vi "Process.vi"(8 "error in":errorcluster, 11 "EmbeddedSMO":refnum<class "SMO.UI.Embedded.lvclass">) -> (0 "error out":errorcluster, 3 "EmbeddedSMO out":refnum<class "SMO.UI.Embedded.lvclass">)   [LabVIEW 2019, in "SMO.UI.Embedded.lvclass"]
doc: "---------------------------------------------------------------\nJKI State Machine Objects™\nhttp://jki.net/state-machine-objects/\nCopyright (C) 2005-2015, JKI <info@jki.net>\nALL RIGHTS RESERVEDJKI State Machine Objects (SMO) 1.0.0.5\nJKI - JKI\nCopyright (c) 2016, JKI"
uses:
  SMO.UI.Embedded.lvclass
  C:/Program Files (x86)/National Instruments/LabVIEW 2019/vi.lib/JKI/JKI SMO/SMO/SMO.lvclass
  C:/Program Files (x86)/National Instruments/LabVIEW 2019/vi.lib/JKI/JKI SMO/SMO.UI/SMO.UI.lvclass
  <vilib>/JKI/JKI SMO/SMO/Typedefs/Parent Call--Enum.ctl
  SMO.UI.Embedded.lvclass/SMO.UI.Embedded.ctl
  <vilib>/JKI/JKI SMO/SMO/SMO.lvclass/SMO.ctl
  <vilib>/JKI/JKI SMO/SMO/Private/ReftoDVR--SMO.vi
  <vilib>/JKI/JKI SMO/SMO.UI/SMO.UI.lvclass
  <vilib>/JKI/JKI SMO/SMO/SMO.lvclass
panel:
  # "For instructions on how to use the JKI State Machine Objects, examples and video tutorials, visit:\nhttp://jki.net/state-machine-objects/\n\nJKI State Machine Objects™\nhttp://jki.net/state-machine-objects/\nCopyright (C) 2005-2015, JKI <info@jki.net>\nALL RIGHTS RESERVED"
  # "SMO UI Template"
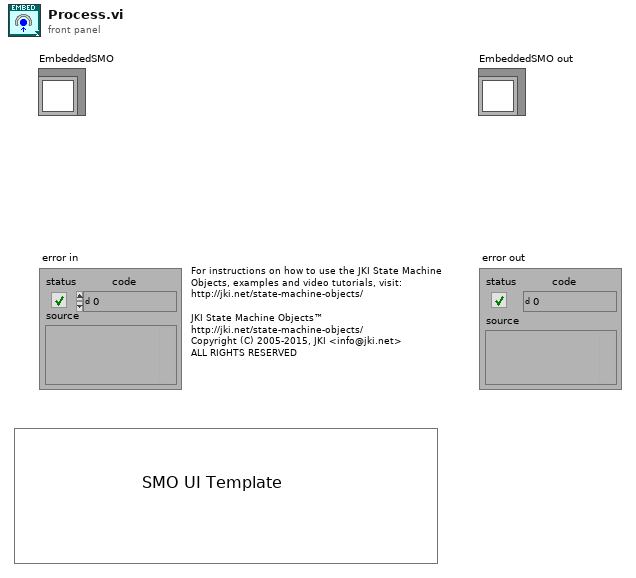
[diagram p1: front panel]
types:
  T1 = typedef "SMO.lvclass/Parent Call--Enum.ctl" = enum16{"Allows parent to run", "Does not request parent to run"}
  T2 = enum32{"invalid app kind", "Development System", "Run Time System", "Student Edition", "Embedded LabVIEW", "Evaluation", "Custom"}
  T3 = enum32{"Invalid", "Standard", "Closed", "Hidden", "Minimized", "Maximized"}
  T4 = typedef "SMO.UI.Embedded.lvclass/PrivateEvents--EmbeddedSMO.WriteName.ctl" = string
  T5 = cluster{"Core":cluster{"Current VI Reference":refnum<vi>, "Close Panel on Exit?":bool, "error":errorcluster}, "Self":refnum<class "SMO.UI.Embedded.lvclass">, "Your string data":string}
  T6 = typedef "SMO.UI.Embedded.lvclass/PrivateEvents--EmbeddedSMO.GetName.ctl" = refnum<notifier>
  T7 = typedef "SMO.UI.Embedded.lvclass/GetUIStateNotifier.ctl" = refnum<notifier>
  T8 = typedef "SMO.UI.Embedded.lvclass/UI State.ctl" = enum16{"unknown", "Opened", "Embedded", "Closed"}
  T9 = typedef "SMO.UI.Embedded.lvclass/PrivateEvents--EmbeddedSMO.GetSubPanelReference.ctl" = refnum<notifier>
  T10 = typedef "SMO.UI.Embedded.lvclass/PrivateEvents--EmbeddedSMO.SetSubpanelReference.ctl" = refnum<vi>
  T11 = cluster{"Current VI Reference":refnum<vi>, "Close Panel on Exit?":bool, "error":errorcluster}
  T12 = typedef "SMO.UI.Embedded.lvclass/PrivateEvents--Cluster.ctl" = cluster{"Get UI State":refnum<user-event>, "SetUIState":refnum<user-event>, "GetSubPanelReference":refnum<user-event>, "SetSubpanelReference":refnum<user-event>, "WriteName":refnum<user-event>, "GetName":refnum<user-event>}
  T13 = typedef "SMO.lvclass/Protected Events.ctl" = cluster{"StopProcesses":refnum<user-event>, "AbortProcesses":refnum<user-event>, "Config Changed":refnum<user-event>, "Dependency":refnum<user-event>}
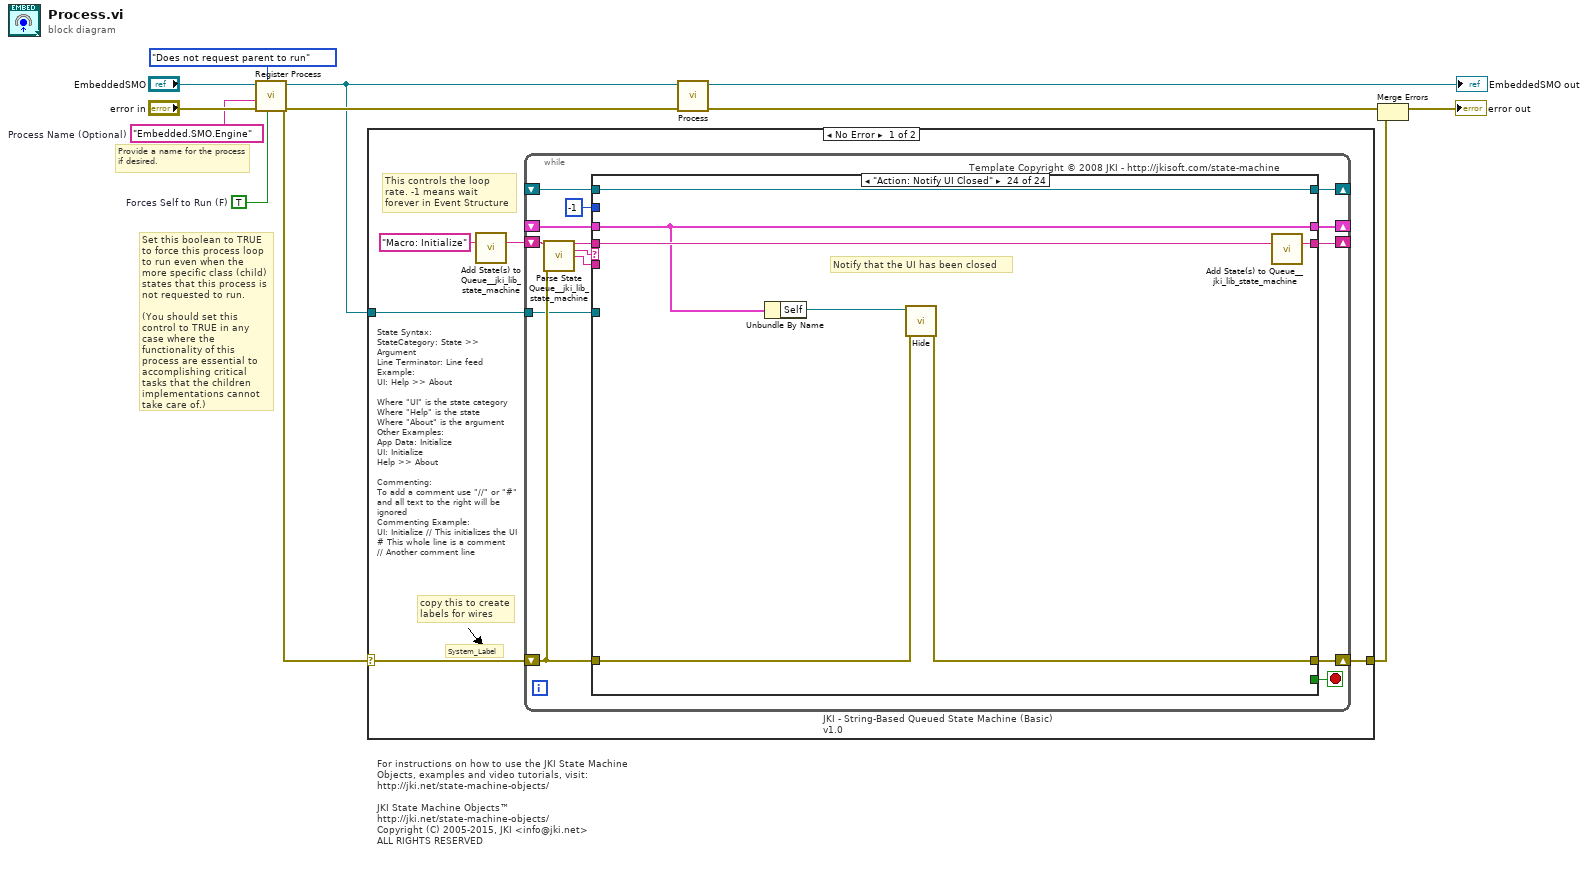
[diagram p0: block diagram]
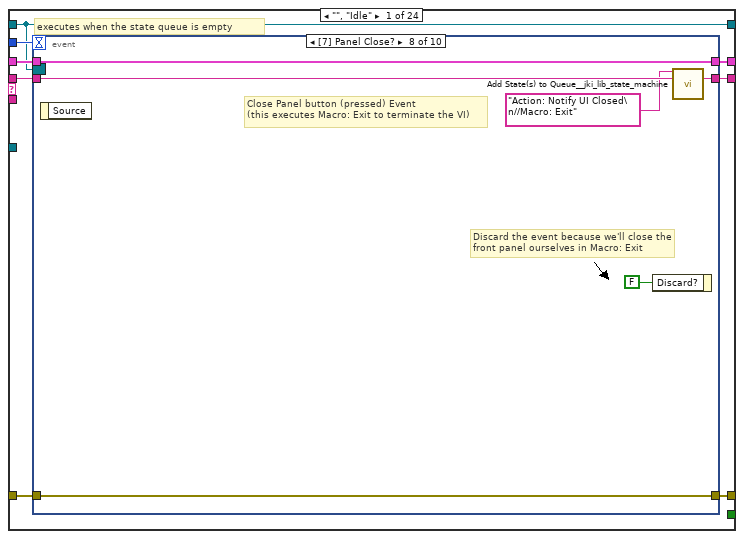
[diagram p2: hidden frame]
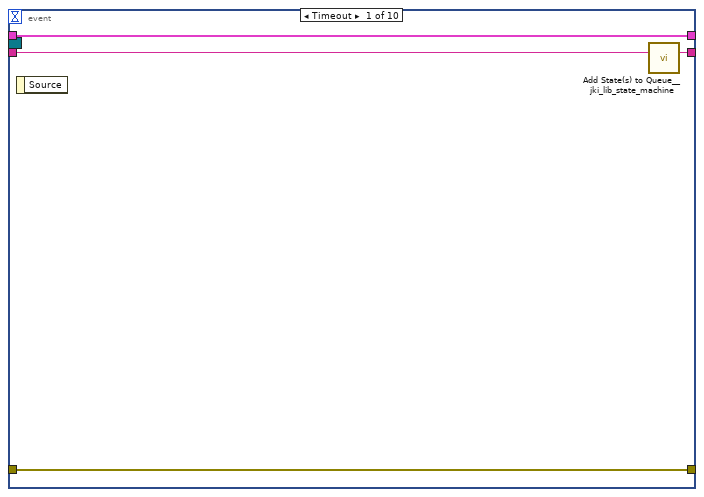
[diagram p3: hidden frame]
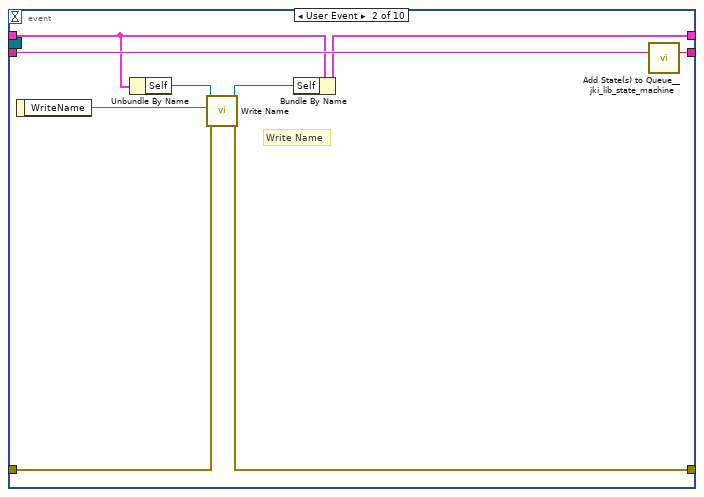
[diagram p4: hidden frame]
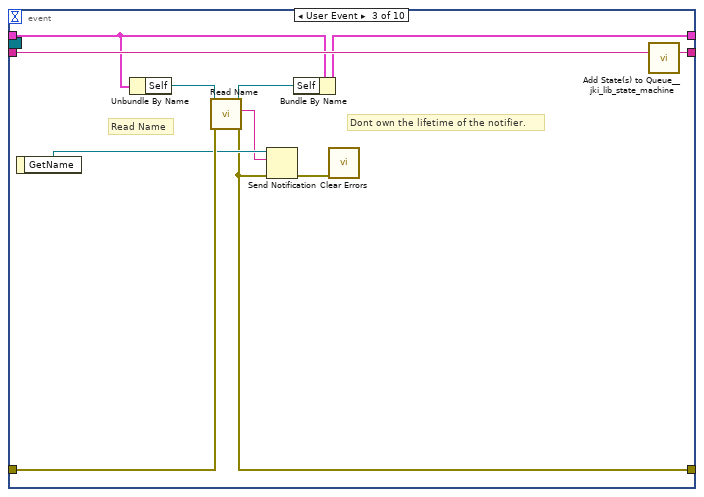
[diagram p5: hidden frame]
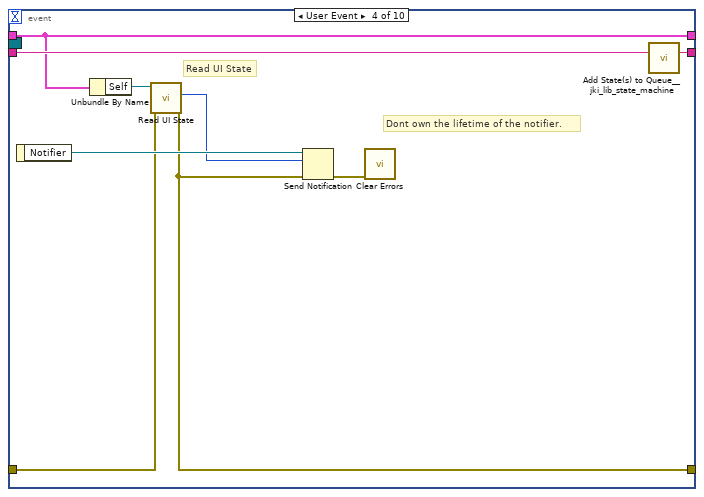
[diagram p6: hidden frame]
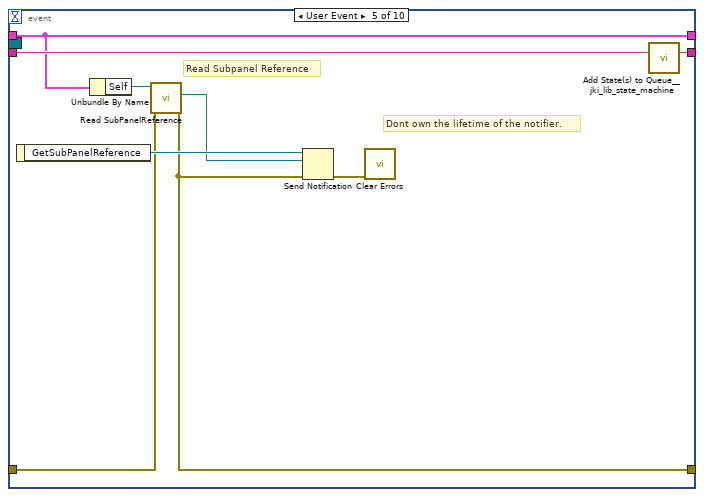
[diagram p7: hidden frame]
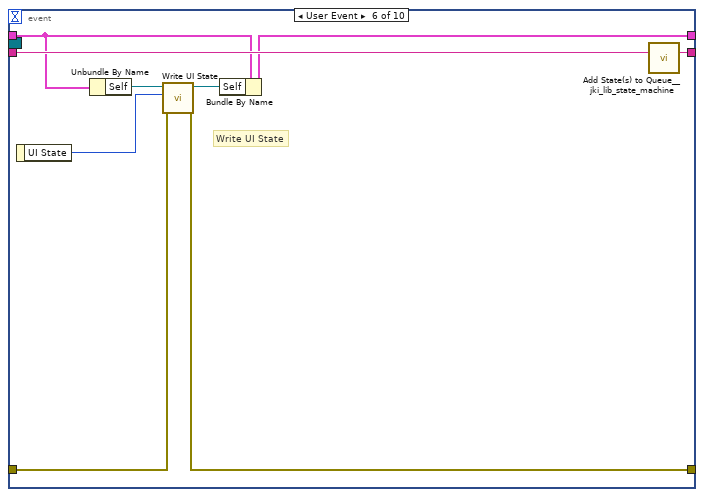
[diagram p8: hidden frame]
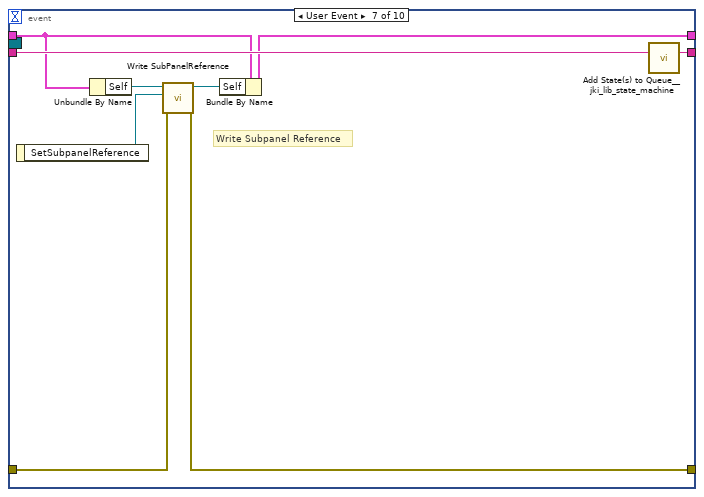
[diagram p9: hidden frame]
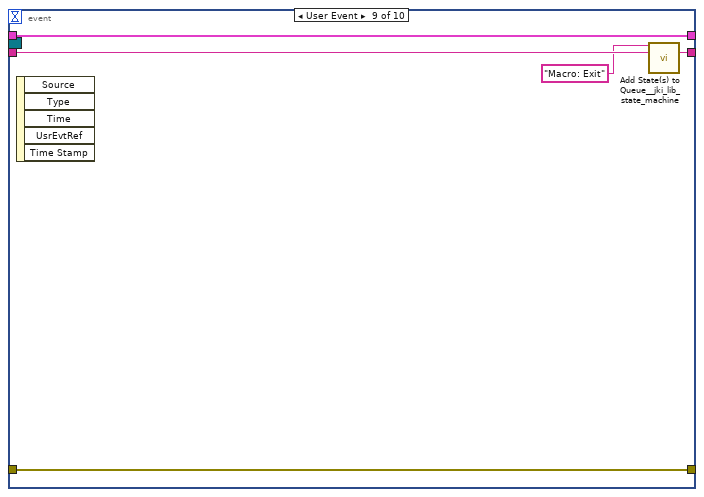
[diagram p10: hidden frame]
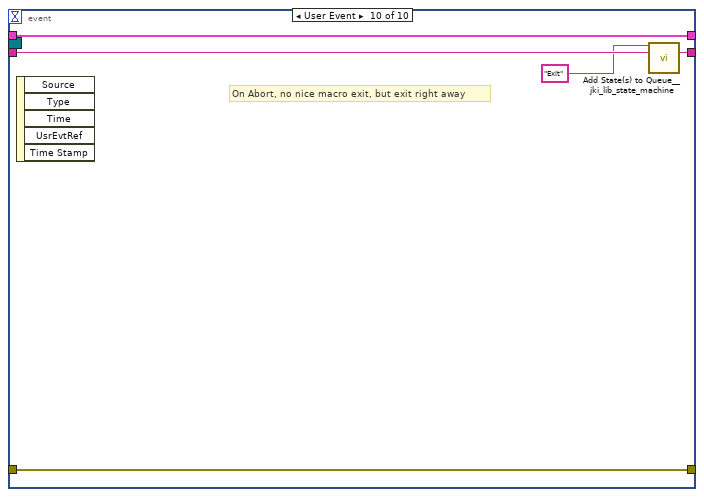
[diagram p11: hidden frame]
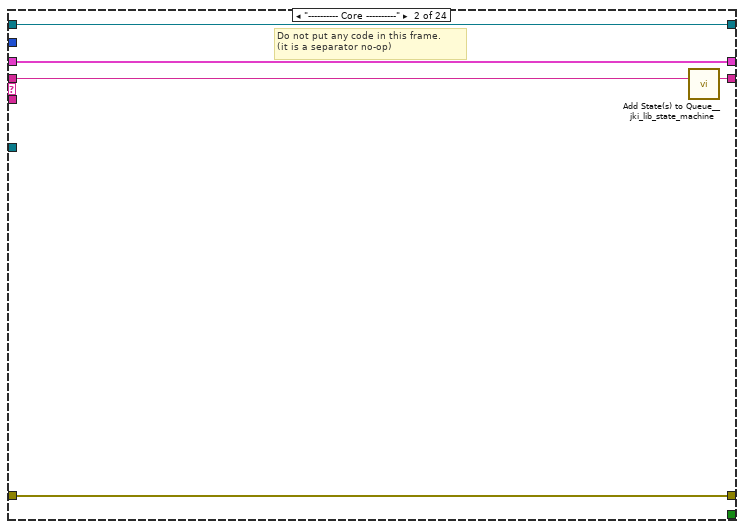
[diagram p12: hidden frame]
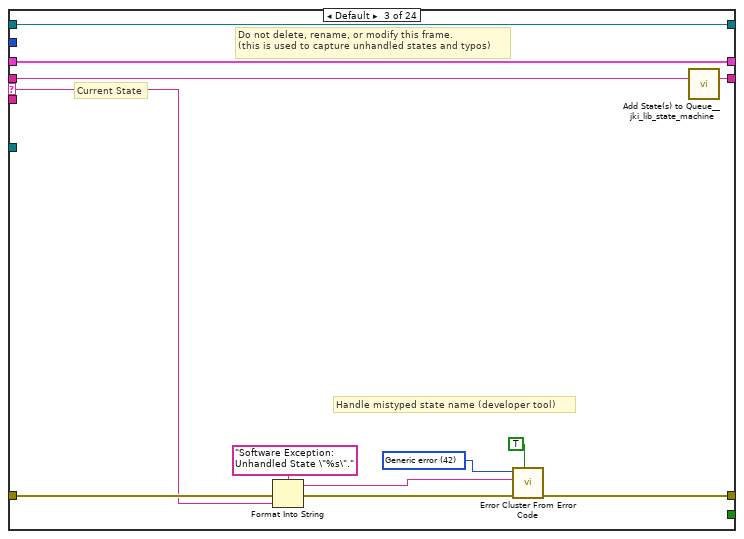
[diagram p13: hidden frame]
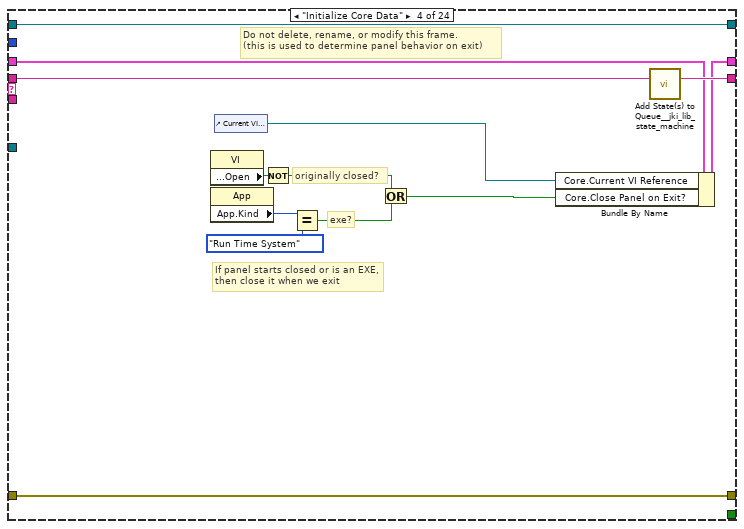
[diagram p14: hidden frame]
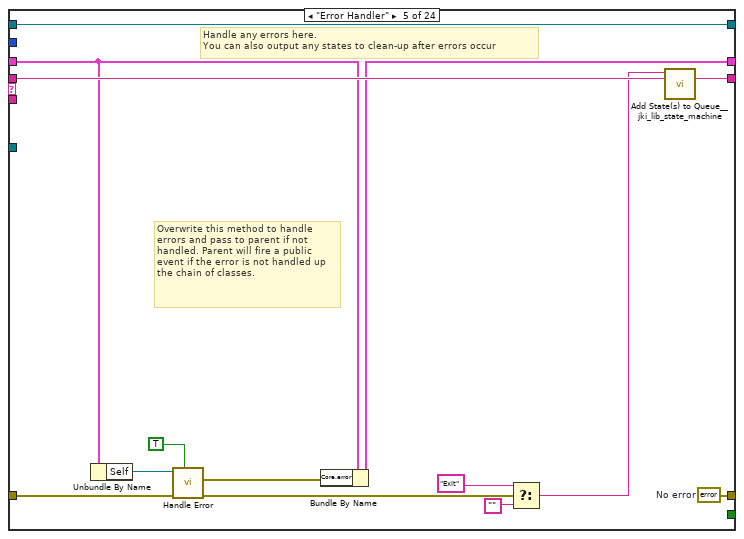
[diagram p15: hidden frame]
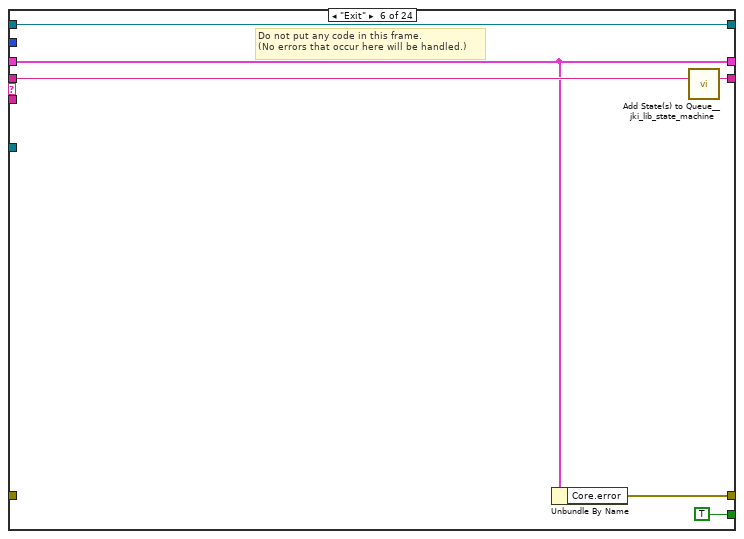
[diagram p16: hidden frame]
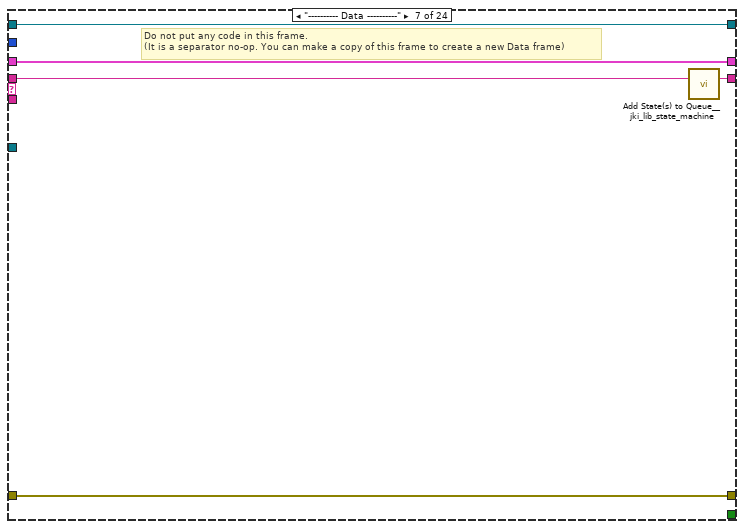
[diagram p17: hidden frame]
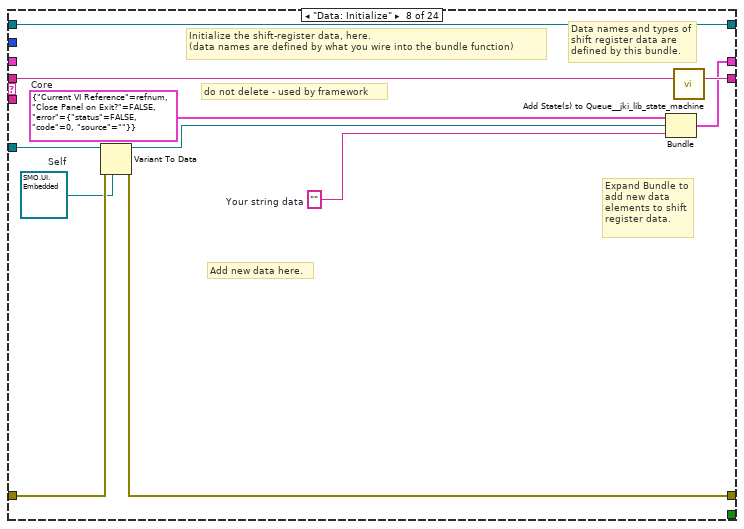
[diagram p18: hidden frame]
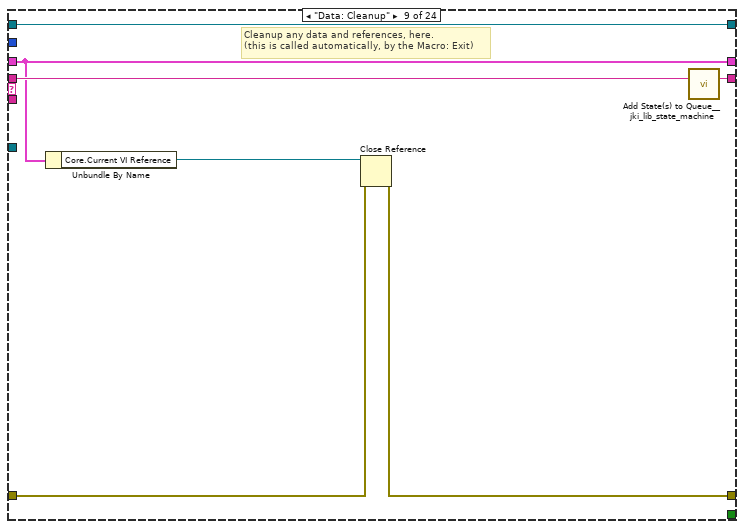
[diagram p19: hidden frame]
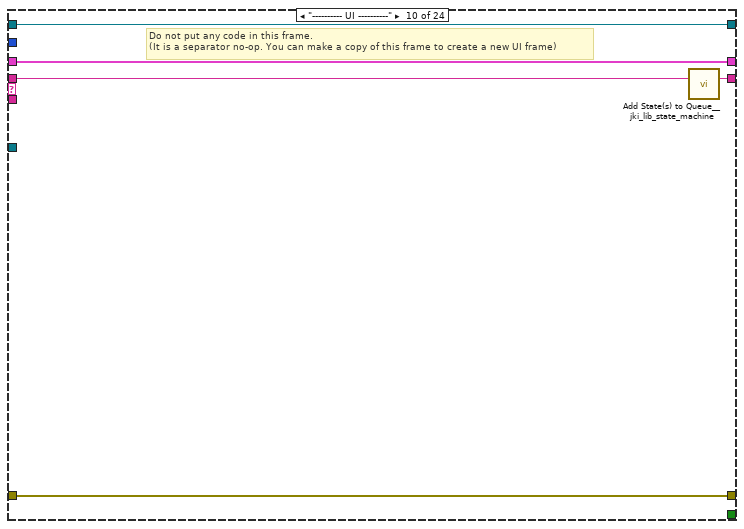
[diagram p20: hidden frame]
diagram:
  w2 = TRUE  # Forces Self to Run (F)
  w1 = "Embedded.SMO.Engine"  # Process Name (Optional)
  # "Provide a name for the process\nif desired."
  # "Set this boolean to TRUE to force this process loop to run even when the more specific class (child) states that this process is not requested to run.\n\n(You should set this control to TRUE in any case where the functionality of this process are essential to accomplishing critical tasks that the children implementations cannot take care of.)"
  # "For instructions on how to use the JKI State Machine Objects, examples and video tutorials, visit:\nhttp://jki.net/state-machine-objects/\n\nJKI State Machine Objects™\nhttp://jki.net/state-machine-objects/\nCopyright (C) 2005-2015, JKI <info@jki.net>\nALL RIGHTS RESERVED"
  n1 = call <vilib>:"Register Process.vi"("Forces Self to Run (F)"=w2, "Parent Call"=Parent_Call--Enum."Does not request parent to run", "error in (no error)"="error in", "Process Name (optional)"=w1, "SMO"="EmbeddedSMO") -> ("error out"=w8:errorcluster, "SMO out"=w7:refnum<class "SMO.UI.Embedded.lvclass">)  [unwired: 5 in]
  n2 = case shown="No Error" w8 {
    selector: w8 -> [w13 w342]
    tunnel: w7 -> [w14 _]
    tunnel: [w12 w342] -> w4
    frame No Error {
      # "State Syntax:\nStateCategory: State >> Argument\nLine Terminator: Line feed\nExample:\nUI: Help >> About\n\nWhere \"UI\" is the state category\nWhere \"Help\" is the state\nWhere \"About\" is the argument\nOther Examples:\nApp Data: Initialize\nUI: Initialize\nHelp >> About\n\nCommenting:\nTo add a comment use \"//\" or \"#\" and all text to the right will be ignored\nCommenting Example:\nUI: Initialize // This initializes the UI\n# This whole line is a comment\n// Another comment line"
      # "copy this to create labels for wires"
      # "This controls the loop rate. -1 means wait forever in Event Structure"
      # "System_Label"
      n3 = call <vilib>:"Add State(s) to Queue__jki_lib_state_machine.vi"("State(s) in (\"\")"="Macro: Initialize") -> ("States Out"=w16:string)  [unwired: 14 in]
      n4 = while "JKI - String-Based Queued State Machine (Basic) v1.0" {
        shift-right: [w23] -> _
        shift-left: _ -> [w22]
        shift-right: [w26] -> w12
        shift-left: w13 -> [w20]
        shift-right: [w25] -> _
        shift-left: w16 -> [w27]
        tunnel: w14 -> [w19]
        shift-right: [w18] -> _
        shift-left: _ -> [w17]
        stop <- w24 stop-if-true
        # "Template Copyright © 2008 JKI - http://jkisoft.com/state-machine"
        n5 = call <vilib>:"Parse State Queue__jki_lib_state_machine.vi"("State Queue"=w27, "Error In (no error)"=w20) -> ("Remaining States"=w29:string, "Current State"=w30:string, "Arguments"=w28:string)  [unwired: 11 in]
        n6 = case shown="\"Action: Notify UI Closed\"" w30 {
          selector: w30 -> [_ _ w121 _ _ _ _ _ _ _ _ _ _ _ _ _ _ _ _ _ _ _ _ _]
          tunnel: w29 -> [w38 w119 w125 w144 w158 w164 w169 w180 w187 w192 w200 w207 w223 w255 w264 w278 w283 w294 w299 w311 w317 w324 w334 w341]
          tunnel: w28 -> [_ _ _ _ _ _ _ _ _ _ _ w201 w217 _ _ _ _ _ _ _ _ _ _ _]
          tunnel: w22 -> [w36 w116 w123 w135 w147 w160 w166 _ w182 w189 w196 w205 w219 w252 w260 w269 w280 w291 w296 w309 w315 w320 w331 w337]
          tunnel: [w35 w117 w127 w141 w149 w159 w167 w175 w183 w190 w198 w202 w220 w253 w262 w276 w281 w285 w297 w304 w312 w321 w325 w335] -> w26
          tunnel: w20 -> [w34 w117 w126 w141 w154 _ w167 w176 w184 w190 w198 w203 w221 w253 w262 w276 w281 w286 w297 w306 w313 w321 w326 w336]
          tunnel: [w37 w118 w124 w143 w157 w163 w168 w179 w186 w191 w199 w206 w222 w254 w263 w277 w282 w293 w298 w310 w316 w323 w333 w340] -> w25
          tunnel: [_ _ _ _ _ TRUE _ _ _ _ _ _ _ _ _ _ _ _ _ _ _ _ _ _] -> w24
          tunnel: [w33 w116 w123 w142 w146 w160 w166 w178 w182 w189 w196 w205 w219 w252 w260 w269 w280 w291 w296 w309 w315 w319 w330 w337] -> w23
          tunnel: -1 ("Timeout") -> [w32 _ _ _ _ _ _ _ _ _ _ _ _ _ _ _ _ _ _ _ _ _ _ _]
          tunnel: w19 -> [_ _ _ _ _ _ _ w173 _ _ _ _ _ _ _ _ _ _ _ _ _ _ _ _]
          tunnel: [w31 w115 w120 w132 w156 w161 w165 w171 w181 w188 w197 w204 w216 w251 w261 w270 w279 w292 w295 w308 w314 w322 w332 w339] -> w18
          tunnel: w17 -> [w31 w115 w120 w132 w156 w161 w165 w171 w181 w188 w197 w204 w216 w251 w261 w270 w279 w292 w295 _ w314 w322 w332 w339]
          frame "", "Idle" {
            # "executes when the state queue is empty"
            n7 = event shown="[7] Panel Close?" {
              selector: w31 -> [_ _ _ _ _ _ _ _ _ _]
              dyn-events: _ -> [_ _ _ _ _ _ _ _ _ _]
              timeout: w32 -> [_ _ _ _ _ _ _ _ _ _]
              tunnel: w38 -> [w42 w51 w62 w71 w80 w89 w98 w104 w109 w114]
              tunnel: [w41 w50 w61 w70 w79 w88 w97 w103 w108 w113] -> w37
              tunnel: w36 -> [w39 w48 w60 w69 w78 w83 w93 w100 w106 w111]
              tunnel: [w40 w45 w52 w63 w72 w84 w94 w99 w107 w112] -> w35
              tunnel: w34 -> [w40 w46 w56 w66 w73 w85 w95 w99 w107 w112]
              tunnel: [w39 w47 w59 w69 w78 w82 w92 w100 w106 w111] -> w33
              event Timeout {
                n8 = event-data() -> ()  [unwired: 1 in, 1 out]
                n9 = call <vilib>:"Add State(s) to Queue__jki_lib_state_machine.vi"("State(s) in (\"\")"=w42) -> ("States Out"=w41:string)  [unwired: 14 in]
              }
              event User Event {
                # "Write Name"
                n10 = event-data() -> ("WriteName"=w49:T4)  [unwired: 1 in]
                n11 = Unbundle By Name(w48) -> ("Self"=w44:refnum<class "SMO.UI.Embedded.lvclass">)
                n12 = call "Write Name.vi"("error in (no error)"=w46, "Name"=w49, "EmbeddedSMO in"=w44) -> ("error out"=w45:errorcluster, "EmbeddedSMO out"=w43:refnum<class "SMO.UI.Embedded.lvclass">)  [unwired: 7 in]
                n13 = Bundle By Name(cluster=w48, "Self"=w43) -> (w47:T5)
                n14 = call <vilib>:"Add State(s) to Queue__jki_lib_state_machine.vi"("State(s) in (\"\")"=w51) -> ("States Out"=w50:string)  [unwired: 14 in]
              }
              event User Event {
                # "Dont own the lifetime of the notifier."
                # "Read Name"
                n15 = event-data() -> ("GetName"=w54:T6)  [unwired: 1 in]
                n16 = Unbundle By Name(w60) -> ("Self"=w58:refnum<class "SMO.UI.Embedded.lvclass">)
                n17 = call "Read Name.vi"("error in (no error)"=w56, "EmbeddedSMO in"=w58) -> ("error out"=w52:errorcluster, "Name"=w53:string, "EmbeddedSMO out"=w57:refnum<class "SMO.UI.Embedded.lvclass">)  [unwired: 7 in]
                n18 = Send Notification(notification=w53, notifier=w54, error in (no error)=w52) -> (error out=w55:errorcluster)  [unwired: 1 out]
                n19 = Bundle By Name(cluster=w60, "Self"=w57) -> (w59:T5)
                n20 = call <vilib>:"Clear Errors.vi"("error in (no error)"=w55) -> ()  [unwired: 5 in, 2 out]
                n21 = call <vilib>:"Add State(s) to Queue__jki_lib_state_machine.vi"("State(s) in (\"\")"=w62) -> ("States Out"=w61:string)  [unwired: 14 in]
              }
              event User Event {
                # "Dont own the lifetime of the notifier."
                # "Read UI State"
                n22 = event-data() -> ("Notifier"=w68:T7)  [unwired: 1 in]
                n23 = Unbundle By Name(w69) -> ("Self"=w67:refnum<class "SMO.UI.Embedded.lvclass">)
                n24 = call "Read UI State.vi"("error in (no error)"=w66, "EmbeddedSMO in"=w67) -> ("error out"=w63:errorcluster, "UI State"=w65:T8)  [unwired: 7 in, 1 out]
                n25 = Send Notification(notification=w65, notifier=w68, error in (no error)=w63) -> (error out=w64:errorcluster)  [unwired: 1 out]
                n26 = call <vilib>:"Clear Errors.vi"("error in (no error)"=w64) -> ()  [unwired: 5 in, 2 out]
                n27 = call <vilib>:"Add State(s) to Queue__jki_lib_state_machine.vi"("State(s) in (\"\")"=w71) -> ("States Out"=w70:string)  [unwired: 14 in]
              }
              event User Event {
                # "Dont own the lifetime of the notifier."
                # "Read Subpanel Reference"
                n28 = event-data() -> ("GetSubPanelReference"=w77:T9)  [unwired: 1 in]
                n29 = Unbundle By Name(w78) -> ("Self"=w75:refnum<class "SMO.UI.Embedded.lvclass">)
                n30 = call "Read SubPanelReference.vi"("error in (no error)"=w73, "EmbeddedSMO in"=w75) -> ("error out"=w72:errorcluster, "SubPanelReference"=w74:refnum<vi>)  [unwired: 7 in, 1 out]
                n31 = Send Notification(notification=w74, notifier=w77, error in (no error)=w72) -> (error out=w76:errorcluster)  [unwired: 1 out]
                n32 = call <vilib>:"Clear Errors.vi"("error in (no error)"=w76) -> ()  [unwired: 5 in, 2 out]
                n33 = call <vilib>:"Add State(s) to Queue__jki_lib_state_machine.vi"("State(s) in (\"\")"=w80) -> ("States Out"=w79:string)  [unwired: 14 in]
              }
              event User Event {
                # "Write UI State"
                n34 = event-data() -> ("UI State"=w86:T8)  [unwired: 1 in]
                n35 = Unbundle By Name(w83) -> ("Self"=w87:refnum<class "SMO.UI.Embedded.lvclass">)
                n36 = call "Write UI State.vi"("error in (no error)"=w85, "UI State"=w86, "EmbeddedSMO in"=w87) -> ("error out"=w84:errorcluster, "EmbeddedSMO out"=w81:refnum<class "SMO.UI.Embedded.lvclass">)  [unwired: 7 in]
                n37 = Bundle By Name(cluster=w83, "Self"=w81) -> (w82:T5)
                n38 = call <vilib>:"Add State(s) to Queue__jki_lib_state_machine.vi"("State(s) in (\"\")"=w89) -> ("States Out"=w88:string)  [unwired: 14 in]
              }
              event User Event {
                # "Write Subpanel Reference"
                n39 = event-data() -> ("SetSubpanelReference"=w90:T10)  [unwired: 1 in]
                n40 = Unbundle By Name(w93) -> ("Self"=w96:refnum<class "SMO.UI.Embedded.lvclass">)
                n41 = call "Write SubPanelReference.vi"("error in (no error)"=w95, "SubPanelReference"=w90, "EmbeddedSMO in"=w96) -> ("error out"=w94:errorcluster, "EmbeddedSMO out"=w91:refnum<class "SMO.UI.Embedded.lvclass">)  [unwired: 7 in]
                n42 = Bundle By Name(cluster=w93, "Self"=w91) -> (w92:T5)
                n43 = call <vilib>:"Add State(s) to Queue__jki_lib_state_machine.vi"("State(s) in (\"\")"=w98) -> ("States Out"=w97:string)  [unwired: 14 in]
              }
              event Panel Close? {
                # "Discard the event because we'll close the front panel ourselves in Macro: Exit"
                # "Close Panel button (pressed) Event\n(this executes Macro: Exit to terminate the VI)"
                n44 = event-data() -> ()  [unwired: 1 in, 1 out]
                n45 = event-data("Discard?"=FALSE) -> ()  [unwired: 1 in, 1 out]
                n46 = call <vilib>:"Add State(s) to Queue__jki_lib_state_machine.vi"("State(s) in Front (\"\")"="Action: Notify UI Closed\n//Macro: Exit", "State(s) in (\"\")"=w104) -> ("States Out"=w103:string)  [unwired: 13 in]
              }
              event User Event {
                n47 = event-data() -> ()  [unwired: 1 in, 5 out]
                n48 = call <vilib>:"Add State(s) to Queue__jki_lib_state_machine.vi"("State(s) in Front (\"\")"="Macro: Exit", "State(s) in (\"\")"=w109) -> ("States Out"=w108:string)  [unwired: 13 in]
              }
              event User Event {
                # "On Abort, no nice macro exit, but exit right away"
                n49 = event-data() -> ()  [unwired: 1 in, 5 out]
                n50 = call <vilib>:"Add State(s) to Queue__jki_lib_state_machine.vi"("State(s) in Front (\"\")"="Exit", "State(s) in (\"\")"=w114) -> ("States Out"=w113:string)  [unwired: 13 in]
              }
            }
          }
          frame "---------- Core ----------" {
            # "Do not put any code in this frame.\n(it is a separator no-op)"
            n51 = call <vilib>:"Add State(s) to Queue__jki_lib_state_machine.vi"("State(s) in (\"\")"=w119) -> ("States Out"=w118:string)  [unwired: 14 in]
          }
          frame Default {
            w130 = 42 items=["No error", "Argument error", "Memory is full", "Out of zone", "End of file", "File already open", "Generic file I/O error", "File not found", "File permission error", "Disk is full", "Duplicate path", "Too many files open", "System feature not enabled", "Resource file not found", "Cannot add resource", "Resource not found", "Image not found", "Image memory error", "Pen does not exist", "Config type invalid", "Config token not found", "Config parse error", "Config memory error", "Bad external code format", "Bad external code offset", "External code not present", "Null window", "Destroy window error", "Null menu", "Print aborted", "Bad print record", "Print driver error", "Windows error during printing", "Memory error during printing", "Print dialog error", "Generic print error", "Invalid device refnum", "Device not found", "Device parameter error", "Device unit error", "Cannot open device", "Device call aborted", "Generic error", "Cancelled by user", "Object ID too low", "Object ID too high", "Object not in heap", "Unknown heap", "Unknown object (invalid DefProc)", "Unknown object (DefProc not in table)", "Message out of range", "Invalid (null) method", "Unknown message", "Manager call not supported", "Bad address", "Network operation in progress", "Network operation timed out", "Connection is busy", "Network attribute not supported", "Network error", "Address in use", "System out of memory", "Connection aborted", "Connection refused", "Not connected", "Already connected", "Connection closed", "Initialization error (interapplication manager)", "Bad occurrence", "Wait on unbound occurrence handler", "Occurrence queue overflow", "Datalog type conflict", "Unused", "Unrecognized type (interapplication manager)", "Memory corrupt", "Failed to make temporary DLL", "Old CIN version", "Drag socket not found", "Failed to load drop-object", "Failed to register OLE object", "Failed to release OLE object", "Format specifier type mismatch", "Unknown format specifier", "Too few format specifiers", "Too many format specifiers", "Scan failed", "Newer CIN version", "Error converting to variant", "Runtime menu error", "Password tampered", "Variant attribute not found", "Incompatible variant data type", "Event data is not available", "Event Store is not present", "Occurrence is not found", "Event Queue is not created", "Event info is not available", "Refnum passed is NULL", "Error retrieving Class GUID", "Error retrieving CoClass GUID", "Error retrieving TypeLib GUID.", "Bad built application magic bytes.", "Specific driver is different from the specific driver associated with the Logical Name.", "There is no session opened to the class driver.", "Max Error", "MAX - Error with config objects", "MAX - Error loading configuration", "MAX - Group not supported"]
            # "Current State"
            # "Do not delete, rename, or modify this frame.\n(this is used to capture unhandled states and typos)"
            # "Handle mistyped state name (developer tool)"
            n52 = Format Into String(format string="Software Exception: Unhandled State \"%s\"." ("message"), error in=w126, w121) -> (resulting string=w129:string, error out=w128:errorcluster)  [unwired: 1 in]
            n53 = call <vilib>:"Error Cluster From Error Code.vi"("show call chain? (False)"=TRUE, "error in (no error)"=w128, "error message (\"\")"=w129, "error code (0)"=w130) -> ("error out"=w127:errorcluster)  [unwired: 5 in]
            n54 = call <vilib>:"Add State(s) to Queue__jki_lib_state_machine.vi"("State(s) in (\"\")"=w125) -> ("States Out"=w124:string)  [unwired: 14 in]
          }
          frame "Initialize Core Data" {
            # "Do not delete, rename, or modify this frame.\n(this is used to determine panel behavior on exit)"
            # "originally closed?"
            # "exe?"
            # "If panel starts closed or is an EXE, then close it when we exit"
            n55 = property class="VI"() -> ("Front Panel.Open"=w140:bool)  [unwired: 2 in, 2 out]
            n56 = property class="App"() -> ("App.Kind"=w139:T2)  [unwired: 2 in, 2 out]
            n57 = control-ref of="Current VI Reference"() -> (w133:refnum<vi>)
            n58 = Not(x=w140) -> (.not. x?=w137:bool)
            n59 = Equal?(x=w139, y=T2."Run Time System" ("Application:Kind")) -> (x = y?=w136:bool)
            n60 = Or(x=w137, y=w136) -> (x .or. y?=w134:bool)
            n61 = Bundle By Name(cluster=w135, "Core.Current VI Reference"=w133, "Core.Close Panel on Exit?"=w134) -> (w142:T5)
            n62 = call <vilib>:"Add State(s) to Queue__jki_lib_state_machine.vi"("State(s) in (\"\")"=w144) -> ("States Out"=w143:string)  [unwired: 14 in]
          }
          frame "Error Handler" {
            w149 = errorcluster {"status"=FALSE, "code"=0, "source"=""}  # No error
            # "Overwrite this method to handle errors and pass to parent if not handled. Parent will fire a public event if the error is not handled up the chain of classes."
            # "Handle any errors here.\nYou can also output any states to clean-up after errors occur"
            n63 = Unbundle By Name(w147) -> ("Self"=w155:refnum<class "SMO.UI.Embedded.lvclass">)
            n64 = call-dynamic "Handle Error.vi"("Stop on Unhandled Error (T)"=TRUE, "error in"=w154, "SMO"=w155) -> ("handling error"=w150:errorcluster, "Unhandled error"=w148:errorcluster)  [unwired: 6 in, 1 out]
            n65 = Bundle By Name(cluster=w147, "Core.error"=w148) -> (w146:T5)
            n66 = Select(t="Exit", s=w150, f="") -> (s? t:f=w151:string)
            n67 = call <vilib>:"Add State(s) to Queue__jki_lib_state_machine.vi"("State(s) in Front (\"\")"=w151, "State(s) in (\"\")"=w158) -> ("States Out"=w157:string)  [unwired: 13 in]
          }
          frame "Exit" {
            # "Do not put any code in this frame.\n(No errors that occur here will be handled.)"
            n68 = Unbundle By Name(w160) -> ("Core.error"=w159:errorcluster)
            n69 = call <vilib>:"Add State(s) to Queue__jki_lib_state_machine.vi"("State(s) in (\"\")"=w164) -> ("States Out"=w163:string)  [unwired: 14 in]
          }
          frame "---------- Data ----------" {
            # "Do not put any code in this frame.\n(It is a separator no-op. You can make a copy of this frame to create a new Data frame)"
            n70 = call <vilib>:"Add State(s) to Queue__jki_lib_state_machine.vi"("State(s) in (\"\")"=w169) -> ("States Out"=w168:string)  [unwired: 14 in]
          }
          frame "Data: Initialize" {
            w170 = T11 {"Current VI Reference"=refnum, "Close Panel on Exit?"=FALSE, "error"={"status"=FALSE, "code"=0, "source"=""}}  # Core
            w174 = refnum<class "SMO.UI.Embedded.lvclass"> refnum  # Self
            w177 = ""  # Your string data
            # "do not delete - used by framework"
            # "Expand Bundle to add new data elements to shift register data."
            # "Add new data here."
            # "Data names and types of shift register data are defined by this bundle."
            # "Initialize the shift-register data, here.\n(data names are defined by what you wire into the bundle function)"
            n71 = Variant To Data(error in=w176, type=w174, Variant=w173) -> (data=w172:refnum<class "SMO.UI.Embedded.lvclass">, error out=w175:errorcluster)
            n72 = Bundle("Core"=w170, "Self"=w172, "Your string data"=w177) -> (w178:T5)  [unwired: 1 in]
            n73 = call <vilib>:"Add State(s) to Queue__jki_lib_state_machine.vi"("State(s) in (\"\")"=w180) -> ("States Out"=w179:string)  [unwired: 14 in]
          }
          frame "Data: Cleanup" {
            # "Cleanup any data and references, here.\n(this is called automatically, by the Macro: Exit)"
            n74 = Unbundle By Name(w182) -> ("Core.Current VI Reference"=w185:refnum<vi>)
            n75 = Close Reference(reference=w185, error in (no error)=w184) -> (error out=w183:errorcluster)
            n76 = call <vilib>:"Add State(s) to Queue__jki_lib_state_machine.vi"("State(s) in (\"\")"=w187) -> ("States Out"=w186:string)  [unwired: 14 in]
          }
          frame "---------- UI ----------" {
            # "Do not put any code in this frame.\n(It is a separator no-op. You can make a copy of this frame to create a new UI frame)"
            n77 = call <vilib>:"Add State(s) to Queue__jki_lib_state_machine.vi"("State(s) in (\"\")"=w192) -> ("States Out"=w191:string)  [unwired: 14 in]
          }
          frame "UI: Initialize" {
            # "Initialize the User Interface, here.\n(this is called automatically, by the Macro: Init)"
            n78 = Unbundle By Name(w196) -> ("Core.Current VI Reference"=w195:refnum<vi>)
            n79 = property class="VI" props=["FP.State"](reference=w195) -> (reference out=w194:refnum<vi>)  [unwired: 1 in, 2 out]
            n80 = invoke class="VI" method="FP.Open"(reference=w194, "State"=T3."Hidden") -> ()  [unwired: 3 in, 5 out]
            n81 = call <vilib>:"Add State(s) to Queue__jki_lib_state_machine.vi"("State(s) in (\"\")"=w200) -> ("States Out"=w199:string)  [unwired: 14 in]
          }
          frame "UI: Cursor Set" {
            # "Argument"
            # "Initialize the User Interface, here.\n(this is called automatically, by the Macro: Init)"
            n82 = disable-structure shown="Default" {
              disable-tunnel: w203 -> [w208 w211]
              disable-tunnel: [w208 w210] -> w202
              disable-tunnel: w201 -> [_ w209]
              frame condition #0 {
              }
              frame condition #1 (active) {
                n83 = case shown="\"Idle\", Default" w209 {
                  tunnel: w211 -> [w213 w215]
                  tunnel: [w212 w214] -> w210
                  frame "Idle", Default {
                    n84 = call <vilib>:"Unset Busy.vi"("error in (no error)"=w213) -> ("error out"=w212:errorcluster)  [unwired: 10 in]
                  }
                  frame "Busy" {
                    n85 = call <vilib>:"Set Busy.vi"("error in (no error)"=w215) -> ("error out"=w214:errorcluster)  [unwired: 9 in, 1 out]
                  }
                }
              }
            }
            n86 = call <vilib>:"Add State(s) to Queue__jki_lib_state_machine.vi"("State(s) in (\"\")"=w207) -> ("States Out"=w206:string)  [unwired: 14 in]
          }
          frame "UI: Front Panel State" {
            # "Argument"
            # "Set Front Panel Open or Closed\n(Usage: \"UI: Front Panel State >> Open|Close\")"
            n87 = Unbundle By Name(w219) -> ("Core.Current VI Reference"=w218:refnum<vi>)
            n88 = disable-structure shown="Default" {
              disable-tunnel: w221 -> [w227 w250]
              disable-tunnel: [w226 w250] -> w220
              disable-tunnel: w218 -> [w225 _]
              disable-tunnel: w217 -> [w224 _]
              frame condition #0 (active) {
                n89 = case shown="\"Open\", Default" w224 {
                  tunnel: w227 -> [w231 w244]
                  tunnel: [w233 w245] -> w226
                  tunnel: w225 -> [w232 w242]
                  frame "Open", Default {
                    n90 = property class="VI"(reference=w232, error in=w231) -> (reference out=w229:refnum<vi>, error out=w230:errorcluster, "FP.State"=w228:T3)
                    n91 = case shown="\"Closed\"" w228 {
                      tunnel: [w236 w239] -> w233
                      tunnel: w230 -> [w235 w239]
                      tunnel: w229 -> [w234 _]
                      frame "Closed" {
                        n92 = invoke class="VI" method="FP.Open"(reference=w234, error in=w235, "Activate"=TRUE, "State"=T3."Standard") -> (error out=w236:errorcluster)  [unwired: 1 in, 4 out]
                      }
                      frame Default {
                      }
                    }
                  }
                  frame "Close" {
                    n93 = property class="VI"(reference=w242, error in=w244) -> (reference out=w241:refnum<vi>, error out=w243:errorcluster, "FP.State"=w240:T3)
                    n94 = case shown="Default" w240 {
                      tunnel: [w246 w249] -> w245
                      tunnel: w243 -> [w246 w248]
                      tunnel: w241 -> [_ w247]
                      frame "Invalid", "Closed" {
                      }
                      frame Default {
                        n95 = invoke class="VI" method="FP.Close"(reference=w247, error in=w248) -> (error out=w249:errorcluster)  [unwired: 1 in, 2 out]
                      }
                    }
                  }
                }
              }
              frame condition #1 {
              }
            }
            n96 = call <vilib>:"Add State(s) to Queue__jki_lib_state_machine.vi"("State(s) in (\"\")"=w223) -> ("States Out"=w222:string)  [unwired: 14 in]
          }
          frame "---------- Macro ----------" {
            # "Do not put any code in this frame.\n(It is a separator no-op. You can make a copy of this frame to create a new Macro frame)"
            n97 = call <vilib>:"Add State(s) to Queue__jki_lib_state_machine.vi"("State(s) in (\"\")"=w255) -> ("States Out"=w254:string)  [unwired: 14 in]
          }
          frame "Macro: Initialize" {
            w258 = "UI: Initialize\nAction: Ready For Info\n//UI: Front Panel State >> Open"  # UI: Initialize Action: Ready For Info //UI: Front Panel State >> Open
            # "Initialization Macro\n(This is called once, when the VI starts)"
            n98 = call <vilib>:"Add State(s) to Queue__jki_lib_state_machine.vi"("State(s) in Front (\"\")"="Data: Initialize\nInitialize Core Data\nEvents: Register", "State(s) in (\"\")"="Process: Sync", "State(s) at Back (\"\")"=w258) -> ("States Out"=w257:string)  [unwired: 12 in]
            n99 = call <vilib>:"Add State(s) to Queue__jki_lib_state_machine.vi"("State(s) in Front (\"\")"=w257, "State(s) in (\"\")"=w264) -> ("States Out"=w263:string)  [unwired: 13 in]
          }
          frame "Macro: Exit" {
            # "Exit Macro\n(This is called once, when the VI exits)"
            n100 = Unbundle By Name(w269) -> ("Core.Close Panel on Exit?"=w275:bool)
            n101 = Select(t="//UI: Front Panel State >> Close", s=w275, f="") -> (s? t:f=w272:string)
            n102 = call <vilib>:"Add State(s) to Queue__jki_lib_state_machine.vi"("State(s) in Front (\"\")"="Data: Cleanup\nEvents: Unregister", "State(s) in (\"\")"="Process: Sync", "State(s) at Back (\"\")"="Exit") -> ("States Out"=w266:string)  [unwired: 12 in]
            n103 = call <vilib>:"Add State(s) to Queue__jki_lib_state_machine.vi"("State(s) in (\"\")"=w272, "State(s) at Back (\"\")"=w266) -> ("States Out"=w271:string)  [unwired: 13 in]
            n104 = call <vilib>:"Add State(s) to Queue__jki_lib_state_machine.vi"("State(s) in Front (\"\")"=w271, "State(s) in (\"\")"=w278) -> ("States Out"=w277:string)  [unwired: 13 in]
          }
          frame "---------- Process ----------" {
            # "Template Separator\n(You can make a copy of, or modify, this frame)"
            n105 = call <vilib>:"Add State(s) to Queue__jki_lib_state_machine.vi"("State(s) in (\"\")"=w283) -> ("States Out"=w282:string)  [unwired: 14 in]
          }
          frame "Process: Sync" {
            n106 = Unbundle By Name(w291) -> ("Self"=w287:refnum<class "SMO.UI.Embedded.lvclass">)
            n107 = call <vilib>:"WaitOnProcessSync.vi"("error in (no error)"=w286, "SMO"=w287) -> ("error out"=w285:errorcluster, "Don't run?"=w290:bool)  [unwired: 7 in, 1 out]
            n108 = Select(t="Data: Cleanup\nEvents: Unregister\nExit", s=w290, f="") -> (s? t:f=w284:string)
            n109 = call <vilib>:"Add State(s) to Queue__jki_lib_state_machine.vi"("State(s) in Front (\"\")"=w284, "State(s) in (\"\")"=w294) -> ("States Out"=w293:string)  [unwired: 13 in]
          }
          frame "---------- Events ----------" {
            # "Template Separator\n(You can make a copy of, or modify, this frame)"
            n110 = call <vilib>:"Add State(s) to Queue__jki_lib_state_machine.vi"("State(s) in (\"\")"=w299) -> ("States Out"=w298:string)  [unwired: 14 in]
          }
          frame "Events: Register" {
            # "Expand to add\nmore events"
            # "Base Class Protected Events"
            n111 = Unbundle By Name(w309) -> ("Self"=w302:refnum<class "SMO.UI.Embedded.lvclass">)
            n112 = call "SMO.UI.Embedded.GetPrivateEvents.vi"("EmbeddedSMO"=w302) -> ("error out"=w300:errorcluster, "Private Events"=w301:T12)  [unwired: 8 in, 1 out]
            n113 = call <vilib>:"GetProtectedEvents.vi"("SMO"=w302) -> ("error out"=w303:errorcluster, "SMO Protected Events"=w307:T13)  [unwired: 8 in, 1 out]
            n114 = register-events(w307, w301) -> (reference out=w308:refnum<event-registration>, error out=w305:errorcluster)  [unwired: 2 in]
            n115 = Merge Errors(w306, w305, w303, w300) -> (w304:errorcluster)
            n116 = call <vilib>:"Add State(s) to Queue__jki_lib_state_machine.vi"("State(s) in (\"\")"=w311) -> ("States Out"=w310:string)  [unwired: 14 in]
          }
          frame "Events: Unregister" {
            n117 = Unregister For Events(event registration refnum=w314, error in=w313) -> (error out=w312:errorcluster)
            n118 = call <vilib>:"Add State(s) to Queue__jki_lib_state_machine.vi"("State(s) in (\"\")"=w317) -> ("States Out"=w316:string)  [unwired: 14 in]
          }
          frame "---------- Action ----------" {
            n119 = Unbundle By Name(w320) -> ("Self"=w318:refnum<class "SMO.UI.Embedded.lvclass">)
            n120 = Bundle By Name(cluster=w320, "Self"=w318) -> (w319:T5)
            n121 = call <vilib>:"Add State(s) to Queue__jki_lib_state_machine.vi"("State(s) in (\"\")"=w324) -> ("States Out"=w323:string)  [unwired: 14 in]
          }
          frame "Action: Ready For Info" {
            n122 = Unbundle By Name(w331) -> ("Self"=w329:refnum<class "SMO.UI.Embedded.lvclass">)
            n123 = call "SMO.UI.Embedded.ReadyForInfo.vi"("error in (no error)"=w326, "ReadyForInfo"=TRUE, "EmbeddedSMO"=w329) -> ("error out"=w325:errorcluster, "EmbeddedSMO out"=w328:refnum<class "SMO.UI.Embedded.lvclass">)  [unwired: 7 in]
            n124 = Bundle By Name(cluster=w331, "Self"=w328) -> (w330:T5)
            n125 = call <vilib>:"Add State(s) to Queue__jki_lib_state_machine.vi"("State(s) in (\"\")"=w334) -> ("States Out"=w333:string)  [unwired: 14 in]
          }
          frame "Action: Notify UI Closed" {
            # "Notify that the UI has been closed"
            n126 = Unbundle By Name(w337) -> ("Self"=w338:refnum<class "SMO.UI.Embedded.lvclass">)
            n127 = call <vilib>:"Hide.vi"("error in (no error)"=w336, "SMO.UI"=w338) -> ("error out"=w335:errorcluster)  [unwired: 8 in, 1 out]
            n128 = call <vilib>:"Add State(s) to Queue__jki_lib_state_machine.vi"("State(s) in (\"\")"=w341) -> ("States Out"=w340:string)  [unwired: 14 in]
          }
        }
      }
    }
    frame Error {
    }
  }
  n129 = call-parent "Process.vi"("error in (no error)"=w8, "SMO.UI"=w7) -> ("error out"=w5:errorcluster, "SMO.UI out"=→"EmbeddedSMO out":refnum<class "SMO.UI.Embedded.lvclass">)  [unwired: 8 in]
  n130 = Merge Errors(w5, w4) -> (→"error out":errorcluster)
